vi "Enum Def.vi"() -> ()   [LabVIEW 2020]
uses:
  Enum type Def.ctl
panel:
  out "Enum 8":T1
  out "Enum 7":T1
  out "Enum 6":T1
  out "Enum 5":T1
  in  "Enum 4":T1
  in  "Enum 3":T1
  in  "Enum 2":T1
  in  "Enum":T1
  # "Make Type Def.      Open type def"
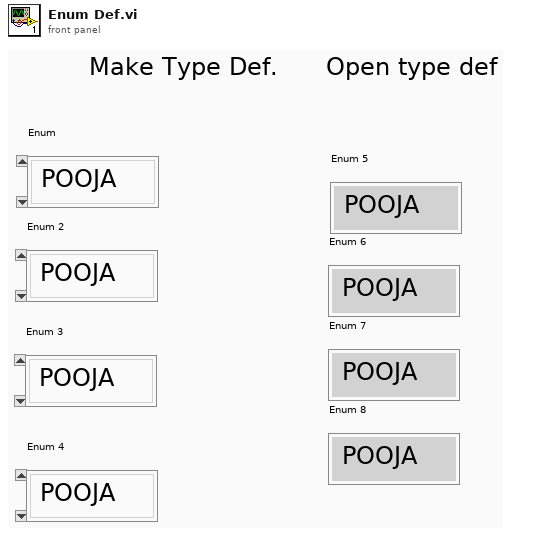
[diagram p1: front panel]
types:
  T1 = typedef "Enum type Def.ctl" = enum16{" POOJA", "don", "Pardeep"}
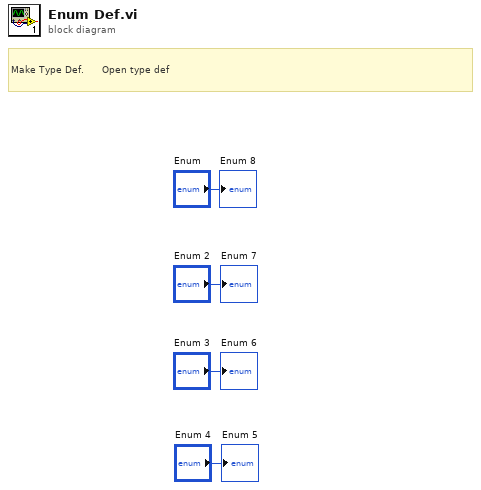
[diagram p0: block diagram]
diagram:
  # "Make Type Def.      Open type def"
  "Enum 5" <- "Enum 4"
  "Enum 6" <- "Enum 3"
  "Enum 7" <- "Enum 2"
  "Enum 8" <- "Enum"
